vi "Read TDMS Data Objects.vi"(8 "error in (no error)":errorcluster, 11 "TDMS-Container in":refnum<class "TDMS-Container.lvclass">) -> (0 "error out":errorcluster, 2 "TDMS Data Objects":refnum<class "TDMS-Data.lvclass">[](array[class]), 3 "TDMS-Container out":refnum<class "TDMS-Container.lvclass">)   [LabVIEW 2014, in "BNT_TDMS.lvlib" / "TDMS-Container.lvclass"]
uses:
  TDMS-Container.lvclass
  TDMSData/TDMS-Data.lvclass
  TDMS-Container.lvclass/TDMS-Container.ctl
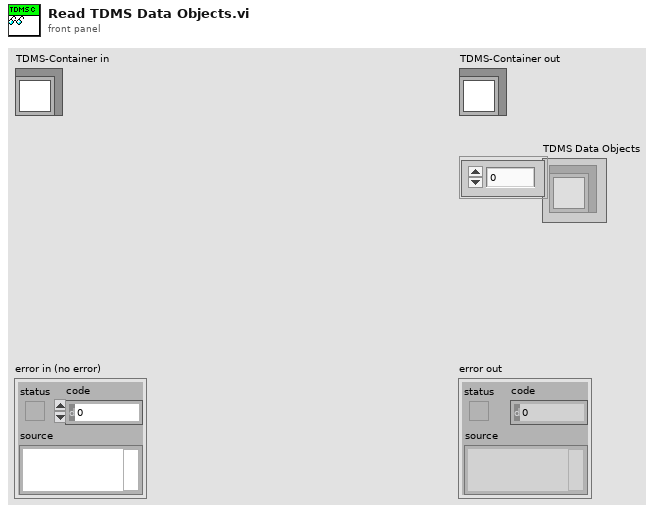
[diagram p1: front panel]
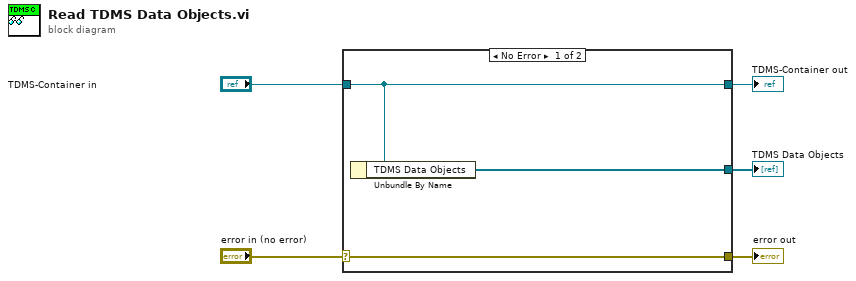
[diagram p0: block diagram]
diagram:
  n1 = case shown="No Error" "error in (no error)" {
    selector: "error in (no error)" -> [w8 w9]
    tunnel: [w8 w9] -> w4
    tunnel: [w7 w10] -> w2
    tunnel: "TDMS-Container in" -> [w7 w10]
    tunnel: [w6 _] -> w1
    frame No Error {
      n2 = Unbundle By Name(w7) -> ("TDMS Data Objects"=w6:refnum<class "TDMS-Data.lvclass">[])
    }
    frame Error {
    }
  }
  "error out" <- w4
  "TDMS-Container out" <- w2
  "TDMS Data Objects" <- w1
